vi "属性对话框.vi"() -> (0 "State":T1={"鼠标进入标题"="", "鼠标离开标题"="", "鼠标进入颜色"=[{"Color Box"=16711680, "Color Box 2"=0}, {"Color Box"=48348, "Color Box 2"=0}], "鼠标离开颜色"=[{"Color Box"=6618880, "Color Box 2"=0}, {"Color Box"=48348, "Color Box 2"=0}]})   [LabVIEW 2011, in "ChangeColorBtn.xctl"]
uses:
  ChangeColorBtn.xctl
  State 1.ctl
panel:
  in  "Tab Control":enum32{"标题", "颜色"}(tab)
  in  "鼠标离开标题":string
  in  "鼠标进入标题":string
  in  "鼠标离开颜色":cluster{"Color Box":u32, "Color Box 2":u32}[](array[cluster]) caption="Array 2"
  in  "鼠标进入颜色":cluster{"Color Box":u32, "Color Box 2":u32}[](array[cluster]) caption="Array"
  in  "stop":bool
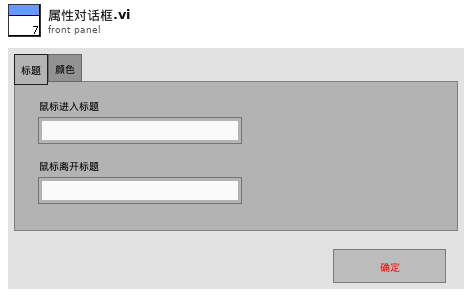
[diagram p1: front panel]
types:
  T1 = typedef "ChangeColorBtn.xctl/State 1.ctl" = cluster{"鼠标进入标题":string, "鼠标离开标题":string, "鼠标进入颜色":cluster{"Color Box":u32, "Color Box 2":u32}[], "鼠标离开颜色":cluster{"Color Box":u32, "Color Box 2":u32}[]}
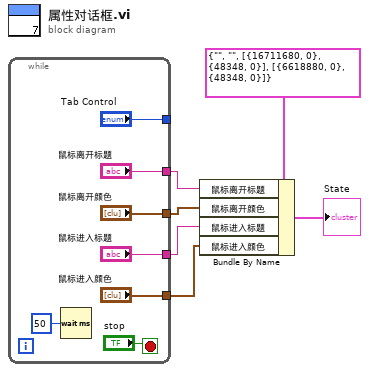
[diagram p0: block diagram]
diagram:
  n1 = while {
    tunnel: ["Tab Control"] -> _
    tunnel: ["鼠标离开标题"] -> w5
    tunnel: ["鼠标离开颜色"] -> w4
    tunnel: ["鼠标进入标题"] -> w3
    tunnel: ["鼠标进入颜色"] -> w2
    stop <- "stop" stop-if-true
    n2 = Wait (ms)(milliseconds to wait=u32 50) -> ()  [unwired: 1 out]
  }
  n3 = Bundle By Name(cluster=T1 {"鼠标进入标题"="", "鼠标离开标题"="", "鼠标进入颜色"=[{"Color Box"=16711680, "Color Box 2"=0}, {"Color Box"=48348, "Color Box 2"=0}], "鼠标离开颜色"=[{"Color Box"=6618880, "Color Box 2"=0}, {"Color Box"=48348, "Color Box 2"=0}]} ("State"), "鼠标离开标题"=w5, "鼠标离开颜色"=w4, "鼠标进入标题"=w3, "鼠标进入颜色"=w2) -> (→"State":T1)
